vi "LeCroy Test Driver - old.vi"() -> ()   [LabVIEW 2013]
doc: "This example shows how to configure the oscilloscope to perform an edge-triggered waveform acquisition."
uses:
  <instrlib>/LeCroy Wave Series/Public/Configure/Configure Edge Trigger.vi
  <instrlib>/LeCroy Wave Series/Public/Data/Read Multiple Waveforms.vi
  <instrlib>/LeCroy Wave Series/LeCroy Wave Series.lvlib
panel:
  in  "Settings":T1={"Ch1"={"On/Off"=FALSE, "Bandwidth (Dropdown)"=0, "Vertical Range (V)"=0.2, "Vertical Offset (V)"=0.0}, "Ch2"={"On/Off"=TRUE, "Bandwidth (Dropdown)"=0, "Vertical Range (V)"=1.2, "Vertical Offset (V)"=0.0}, "Ch3"={"On/Off"=TRUE, "Bandwidth (Dropdown)"=0, "Vertical Range (V)"=0.2, "Vertical Offset (V)"=0.0}, "Ch4"={"On/Off"=FALSE, "Bandwidth (Dropdown)"=0, "Vertical Range (V)"=0.2, "Vertical Offset (V)"=0.0}, "LeCroy IP"="169.254.20.90", "T axis"={"Time base (s/div)"=0.0002, "Time offset (s)"=0.0, "Max Sample Points"=5000}, "Trig"={"Trigger mode"=2, "Trigger Slope"=0, "Trigger Source"=1, "Trigger Level (V)"=0.04}} {"Trig"."Trigger mode" items=["Auto", "Normal", "Single", "Single, auto trigger"]; "Trig"."Trigger Slope" items=["Rising", "Falling"]; "Trig"."Trigger Source" items=["Channel 1", "Channel 2", "Channel 3", "Channel 4", "External", "Power Line"]; "Trig"."Trigger Level (V)" format="%#_6p"; "T axis"."Max Sample Points" format="%.0p" items=["50"=50, "100"=100, "250"=250, "500"=500, "1000"=1000, "2500"=2500, "5K"=5000, "10K"=10000, "25K"=25000, "50K"=50000, "100K"=100000, "250K"=250000, "500K"=500000, "1M"=1000000, "2M"=2000000, "2.5M"=2500000, "5M"=5000000, "10M"=10000000, "25M"=25000000, "50M"=50000000, "100M"=100000000]; "T axis"."Time base (s/div)" format="%#_6p"; "Ch4"."Bandwidth (Dropdown)" items=["Full", "20MHZ", "25MHZ", "200MHZ", "250MHZ", "1GHZ", "3GHZ", "4GHZ"]; "Ch3"."Bandwidth (Dropdown)" items=["Full", "20MHZ", "25MHZ", "200MHZ", "250MHZ", "1GHZ", "3GHZ", "4GHZ"]; "Ch2"."Bandwidth (Dropdown)" items=["Full", "20MHZ", "25MHZ", "200MHZ", "250MHZ", "1GHZ", "3GHZ", "4GHZ"]; "Ch1"."Bandwidth (Dropdown)" items=["Full", "20MHZ", "25MHZ", "200MHZ", "250MHZ", "1GHZ", "3GHZ", "4GHZ"]}
  out "Aquire waveform time (ms)":u32
  out "Waveform Data":waveform(dbl)[](graph)
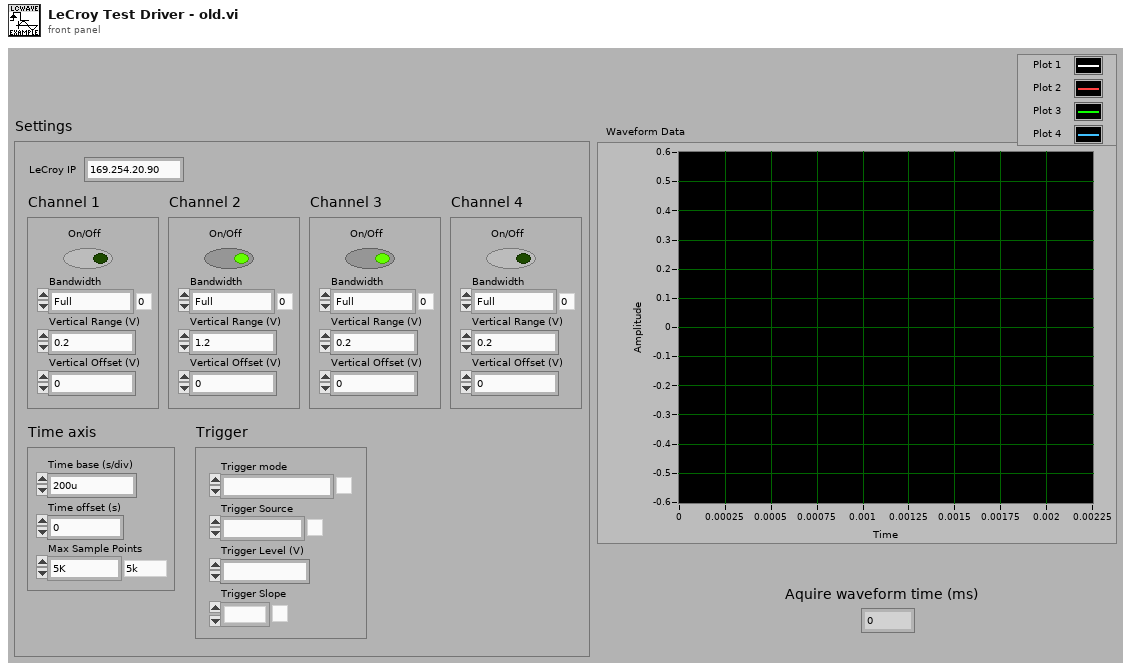
[diagram p1: front panel]
types:
  T1 = cluster{"Ch1":cluster{"On/Off":bool, "Bandwidth (Dropdown)":u16, "Vertical Range (V)":dbl, "Vertical Offset (V)":dbl}, "Ch2":cluster{"On/Off":bool, "Bandwidth (Dropdown)":u16, "Vertical Range (V)":dbl, "Vertical Offset (V)":dbl}, "Ch3":cluster{"On/Off":bool, "Bandwidth (Dropdown)":u16, "Vertical Range (V)":dbl, "Vertical Offset (V)":dbl}, "Ch4":cluster{"On/Off":bool, "Bandwidth (Dropdown)":u16, "Vertical Range (V)":dbl, "Vertical Offset (V)":dbl}, "LeCroy IP":string, "T axis":cluster{"Time base (s/div)":dbl, "Time offset (s)":dbl, "Max Sample Points":i32}, "Trig":cluster{"Trigger mode":u16, "Trigger Slope":u16, "Trigger Source":u16, "Trigger Level (V)":dbl}}
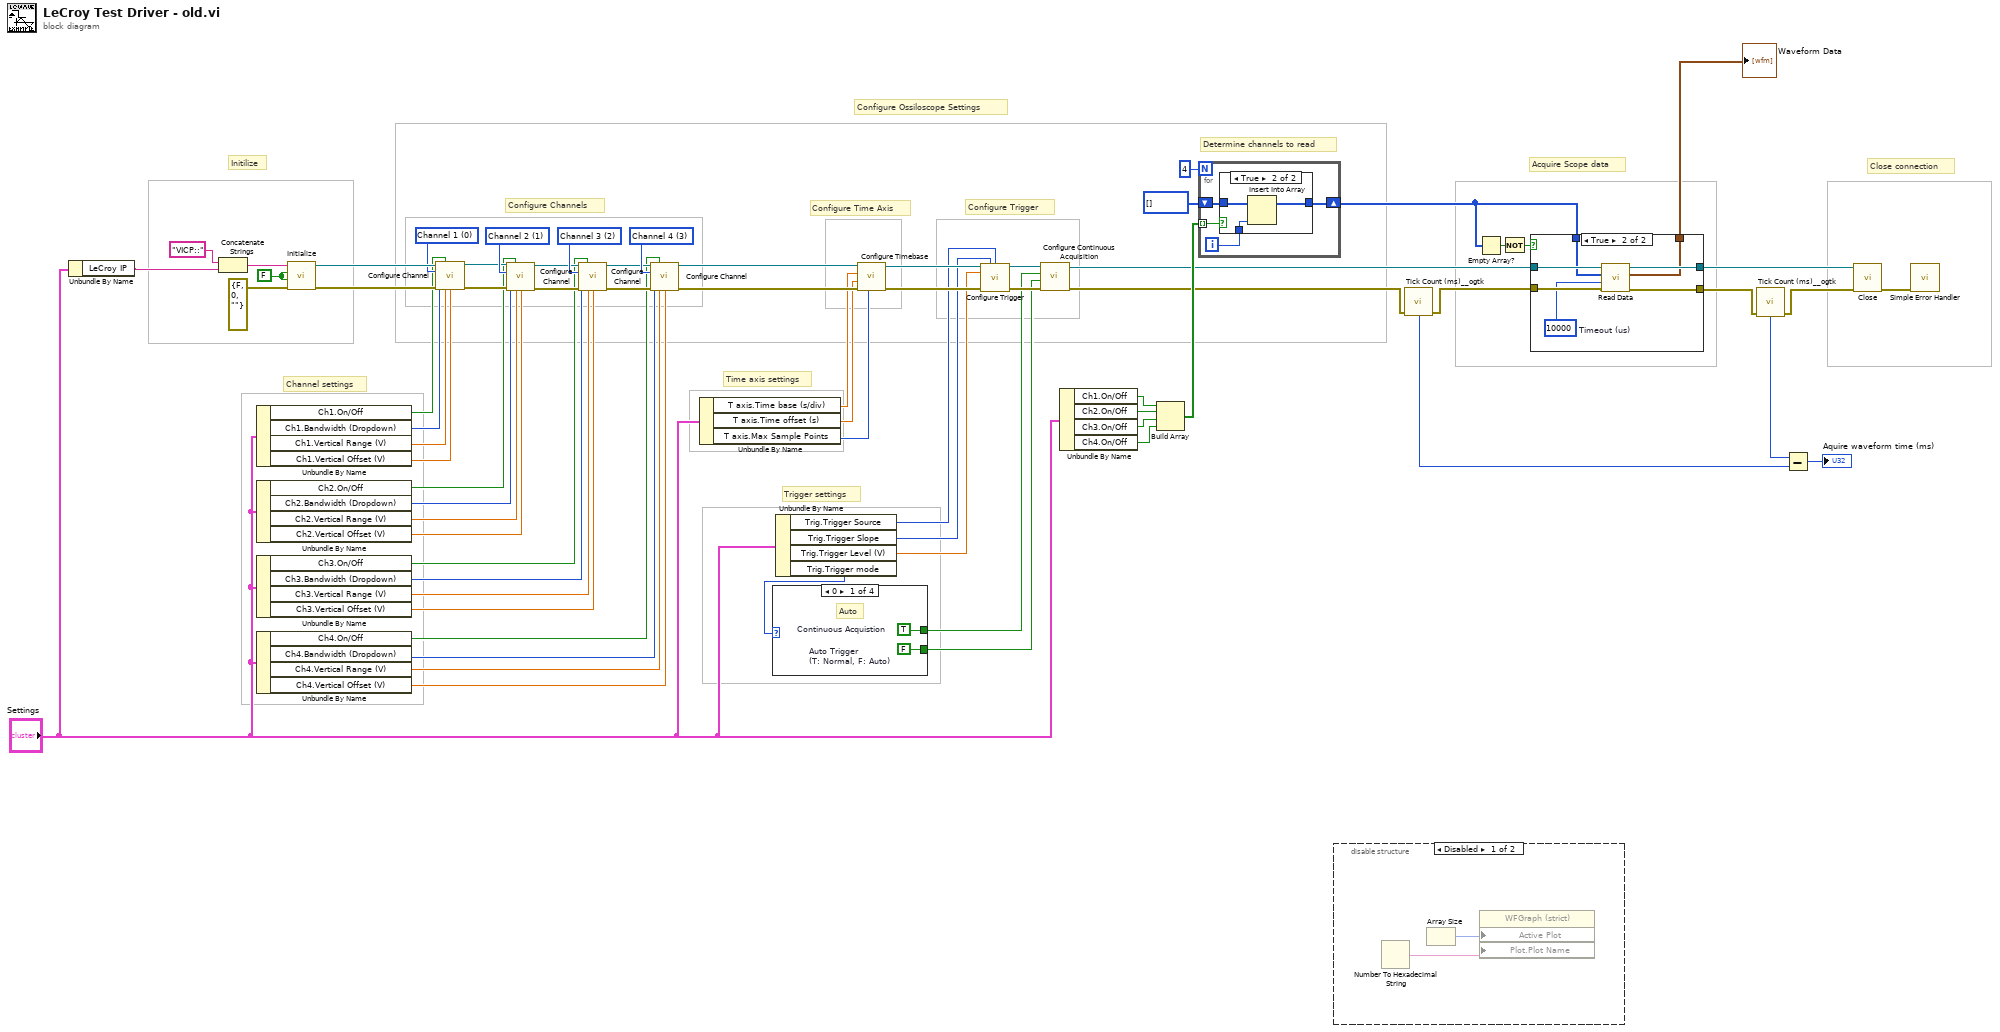
[diagram p0: block diagram]
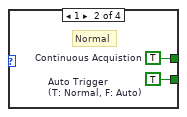
[diagram p5: hidden frame]
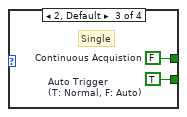
[diagram p6: hidden frame]
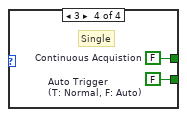
[diagram p7: hidden frame]
diagram:
  w60 = u16 3 items=["Channel 1", "Channel 2", "Channel 3", "Channel 4"] ("Source (0: Channel 1)")
  w61 = u16 2 items=["Channel 1", "Channel 2", "Channel 3", "Channel 4"] ("Source (0: Channel 1)")
  w62 = u16 1 items=["Channel 1", "Channel 2", "Channel 3", "Channel 4"] ("Source (0: Channel 1)")
  w63 = u16 0 items=["Channel 1", "Channel 2", "Channel 3", "Channel 4"] ("Source (0: Channel 1)")
  w67 = FALSE ("Reset? (T: Yes)")
  # "Close connection"
  # "Acquire Scope data"
  # "Determine channels to read"
  # "Trigger settings"
  # "Configure Trigger"
  # "Configure Time Axis"
  # "Time axis settings"
  # "Channel settings"
  # "Configure Channels"
  # "Configure Ossiloscope Settings"
  # "Initilize"
  n1 = Unbundle By Name("Settings") -> ("LeCroy IP"=w18:string)
  n2 = Concatenate Strings("VICP::", w18) -> (w65:string)
  n3 = Unbundle By Name("Settings") -> ("Ch1.On/Off"=w31:bool, "Ch1.Bandwidth (Dropdown)"=w36:u16, "Ch1.Vertical Range (V)"=w37:dbl, "Ch1.Vertical Offset (V)"=w38:dbl)
  n4 = Unbundle By Name("Settings") -> ("Ch2.On/Off"=w28:bool, "Ch2.Bandwidth (Dropdown)"=w29:u16, "Ch2.Vertical Range (V)"=w30:dbl, "Ch2.Vertical Offset (V)"=w27:dbl)
  n5 = Unbundle By Name("Settings") -> ("Ch3.On/Off"=w22:bool, "Ch3.Bandwidth (Dropdown)"=w21:u16, "Ch3.Vertical Range (V)"=w20:dbl, "Ch3.Vertical Offset (V)"=w19:dbl)
  n6 = Unbundle By Name("Settings") -> ("Ch4.On/Off"=w24:bool, "Ch4.Bandwidth (Dropdown)"=w25:u16, "Ch4.Vertical Range (V)"=w26:dbl, "Ch4.Vertical Offset (V)"=w23:dbl)
  n7 = call <instrlib>:"Initialize.vi"("error in (no error)"=errorcluster {"status"=FALSE, "code"=0, "source"=""}, "Reset? (T: Yes)"=w67, "ID Query? (T: Yes)"=w67, "VISA resource name"=w65) -> ("error out"=w68:errorcluster, "VISA resource name out"=w69:refnum<visa-resource-name>)  [unwired: 6 in]
  n8 = call <instrlib>:"Configure Channel.vi"("VISA resource name"=w69, "Enable Channel (T:On)"=w31, "Bandwidth (0: Full)"=w36, "Channel (0: Channel 1)"=w63, "error in (no error)"=w68, "Vertical Range (10.0 V)"=w37, "Vertical Offset (0.0 V)"=w38) -> ("VISA resource name out"=w59:refnum<visa-resource-name>, "error out"=w58:errorcluster)  [unwired: 7 in]
  n9 = call <instrlib>:"Configure Channel.vi"("VISA resource name"=w59, "Enable Channel (T:On)"=w28, "Bandwidth (0: Full)"=w29, "Channel (0: Channel 1)"=w62, "error in (no error)"=w58, "Vertical Range (10.0 V)"=w30, "Vertical Offset (0.0 V)"=w27) -> ("VISA resource name out"=w56:refnum<visa-resource-name>, "error out"=w57:errorcluster)  [unwired: 7 in]
  n10 = call <instrlib>:"Configure Channel.vi"("VISA resource name"=w56, "Enable Channel (T:On)"=w22, "Bandwidth (0: Full)"=w21, "Channel (0: Channel 1)"=w61, "error in (no error)"=w57, "Vertical Range (10.0 V)"=w20, "Vertical Offset (0.0 V)"=w19) -> ("VISA resource name out"=w55:refnum<visa-resource-name>, "error out"=w54:errorcluster)  [unwired: 7 in]
  n11 = call <instrlib>:"Configure Channel.vi"("VISA resource name"=w55, "Enable Channel (T:On)"=w24, "Bandwidth (0: Full)"=w25, "Channel (0: Channel 1)"=w60, "error in (no error)"=w54, "Vertical Range (10.0 V)"=w26, "Vertical Offset (0.0 V)"=w23) -> ("VISA resource name out"=w53:refnum<visa-resource-name>, "error out"=w52:errorcluster)  [unwired: 7 in]
  n12 = Unbundle By Name("Settings") -> ("T axis.Time base (s/div)"=w17:dbl, "T axis.Time offset (s)"=w16:dbl, "T axis.Max Sample Points"=w15:i32)
  n13 = Unbundle By Name("Settings") -> ("Trig.Trigger Source"=w6:u16, "Trig.Trigger Slope"=w5:u16, "Trig.Trigger Level (V)"=w4:dbl, "Trig.Trigger mode"=w2:u16)
  n14 = case shown="0" w2 {
    tunnel: [w72 w74 w76 w78] -> w7
    tunnel: [w71 w73 w75 w77] -> w8
    frame 0 {
      w71 = FALSE  # Auto Trigger (T: Normal, F: Auto)
      w72 = TRUE  # Continuous Acquistion
      # "Auto"
    }
    frame 1 {
      w73 = TRUE  # Auto Trigger (T: Normal, F: Auto)
      w74 = TRUE  # Continuous Acquistion
      # "Normal"
    }
    frame 2, Default {
      w75 = TRUE  # Auto Trigger (T: Normal, F: Auto)
      w76 = FALSE  # Continuous Acquistion
      # "Single"
    }
    frame 3 {
      w77 = FALSE  # Auto Trigger (T: Normal, F: Auto)
      w78 = FALSE  # Continuous Acquistion
      # "Single"
    }
  }
  n15 = call <instrlib>:"Configure Timebase.vi"("Maximum Sample Points (500)"=w15, "error in (no error)"=w52, "Position (0.0 s)"=w16, "Timebase (0.0005 s)"=w17, "VISA resource name"=w53) -> ("error out"=w11:errorcluster, "VISA resource name out"=w14:refnum<visa-resource-name>)  [unwired: 5 in]
  n16 = call-poly <instrlib>:"Configure Trigger.vi"("VISA resource name"=w14, "Trigger Slope (0: Rising)"=w5, "Trigger Source (0: Channel 1)"=w6, "Trigger Level (0.0 V)"=w4, "error in (no error)"=w11) -> ("VISA resource name out"=w13:refnum<visa-resource-name>, "error out"=w12:errorcluster)  [unwired: 9 in]
  n17 = call <instrlib>:"Configure Continuous Acquisition.vi"("error in (no error)"=w12, "Auto Trigger Enabled (T: Normal)"=w8, "Continuous Acquisition Mode (T: On)"=w7, "VISA resource name"=w13) -> ("error out"=w10:errorcluster, "VISA resource name out"=w9:refnum<visa-resource-name>)  [unwired: 6 in]
  n18 = Unbundle By Name("Settings") -> ("Ch1.On/Off"=w35:bool, "Ch2.On/Off"=w34:bool, "Ch3.On/Off"=w33:bool, "Ch4.On/Off"=w32:bool)
  n19 = Build Array(w35, w34, w33, w32) -> (w51:bool[])
  n20 = for {
    N: 4 -> [_]
    tunnel: w51 -> [w79] mode=indexing
    shift-right: [w80] -> w46
    shift-left: i32[] [] -> [w81]
    i -> [w82]
    n21 = case shown="True" w79 {
      tunnel: w82 -> [_ w86]
      tunnel: w81 -> [w83 w85]
      tunnel: [w83 w84] -> w80
      frame False {
      }
      frame True {
        n22 = Insert Into Array(array=w85, new element=w86) -> (w84:i32[])  [unwired: 1 in]
      }
    }
  }
  n23 = disable-structure shown="Disabled" {
    frame Disabled {
      n24 = Number To Hexadecimal String() -> (0:w88:string)  [unwired: 2 in]
      n25 = Array Size() -> (size(s)=w87:i32)  [unwired: 1 in]
      n26 = property on="Property Node" class="WFGraph (strict)"("Active Plot"=w87, "Plot.Plot Name"=w88) -> ()  [unwired: 2 in, 2 out]
    }
    frame Enabled {
    }
  }
  n27 = call <userlib>:"Tick Count (ms)__ogtk.vi"("error in (no error)"=w10) -> ("error out"=w43:errorcluster, "millisecond timer value"=w40:u32)  [unwired: 9 in]
  n28 = Empty Array?(array=w46) -> (empty?=w45:bool)
  n29 = Not(x=w45) -> (.not. x?=w44:bool)
  n30 = case shown="True" w44 {
    tunnel: [w90 w97] -> w48
    tunnel: w9 -> [w90 w96]
    tunnel: w43 -> [w89 w95]
    tunnel: [w89 w94] -> w1
    tunnel: [_ w93] -> w47
    tunnel: w46 -> [_ w91]
    frame False {
    }
    frame True {
      w92 = u32 10000  # Timeout (us)
      n31 = call-poly <instrlib>:"Read Data.vi"("error in (no error)"=w95, "Timeout (10000 ms)"=w92, "Channels"=w91, "VISA resource name"=w96) -> ("error out"=w94:errorcluster, "Waveform Data"=w93:waveform(dbl)[], "VISA resource name out"=w97:refnum<visa-resource-name>)  [unwired: 5 in]
    }
  }
  "Waveform Data" <- w47
  n32 = call <userlib>:"Tick Count (ms)__ogtk.vi"("error in (no error)"=w1) -> ("error out"=w42:errorcluster, "millisecond timer value"=w41:u32)  [unwired: 9 in]
  n33 = Subtract(x=w41, y=w40) -> (x-y=→"Aquire waveform time (ms)":u32)
  n34 = call <instrlib>:"Close.vi"("error in (no error)"=w42, "VISA resource name"=w48) -> ("error out"=w70:errorcluster)  [unwired: 9 in]
  n35 = call <vilib>:"Simple Error Handler.vi"("error in (no error)"=w70) -> ()  [unwired: 4 in, 5 out]
